vi "SP Read Array.vi"(8 "error in":errorcluster, 11 "Pressure Setpoint in":refnum<class "Pressure Setpoint.lvclass">) -> (0 "error out":errorcluster, 1 "Changed or First Call?":bool, 2 "Pressure SP":dbl[](array[numeric]), 3 "Pressure Setpoint out":refnum<class "Pressure Setpoint.lvclass">)   [LabVIEW 2023, in "Pressure Setpoint.lvclass"]
uses:
  Pressure Setpoint.lvclass
  Parents/Setpoint/Setpoint.lvclass
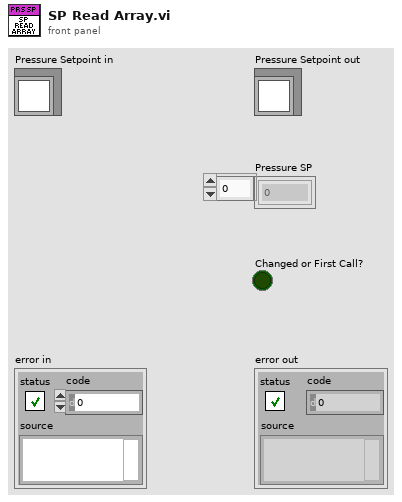
[diagram p1: front panel]
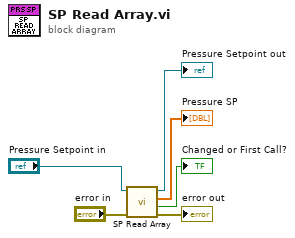
[diagram p0: block diagram]
diagram:
  n1 = call-parent "SP Read Array.vi"("error in"="error in", "Setpoint in"="Pressure Setpoint in") -> ("error out"=→"error out":errorcluster, "Changed or First Call?"=→"Changed or First Call?":bool, "Current Setpoint"=→"Pressure SP":dbl[], "Setpoint out"=→"Pressure Setpoint out":refnum<class "Pressure Setpoint.lvclass">)  [unwired: 6 in]
